vi "Pololu.Pololu Value to Deg and us Converter.vi"(7 "us to Units Mult":dbl=4.0, 9 "Pololu Value":u16, 11 "Range Info":T1={"Min us"=500.0, "Max us"=2500.0, "Min deg"=0.0, "Max deg"=270.0, "LStopDeg"=0.0, "UStopDeg"=270.0}) -> (1 "Pos (Deg)":dbl max=270.0, 3 "Pos (us)":dbl max=270.0)   [LabVIEW 2018]
uses:
  Pololu.Device Range Config.ctl
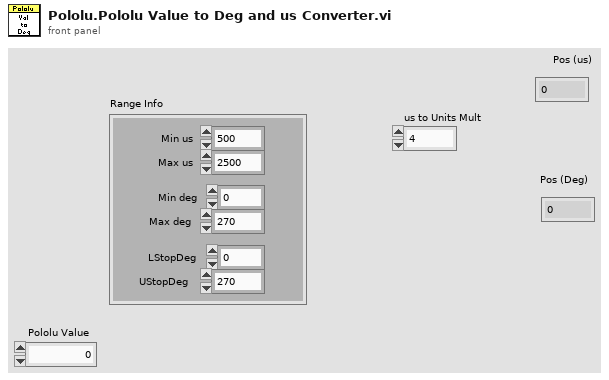
[diagram p1: front panel]
types:
  T1 = typedef "Pololu.Device Range Config.ctl" = cluster{"Min us":dbl, "Max us":dbl, "Min deg":dbl, "Max deg":dbl, "LStopDeg":dbl, "UStopDeg":dbl}
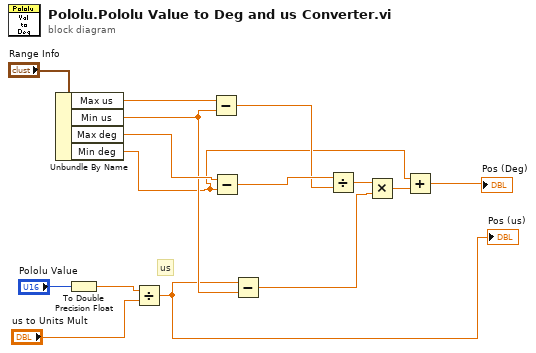
[diagram p0: block diagram]
diagram:
  # "us"
  n1 = Unbundle By Name("Range Info") -> ("Max us"=w10:dbl, "Min us"=w6:dbl, "Max deg"=w11:dbl, "Min deg"=w3:dbl)
  n2 = To Double Precision Float(number="Pololu Value") -> (double precision float=w8:dbl)
  n3 = Divide(x=w8, y="us to Units Mult") -> (x/y=w1:dbl)
  "Pos (us)" <- w1
  n4 = Subtract(x=w10, y=w6) -> (x-y=w4:dbl)
  n5 = Subtract(x=w11, y=w3) -> (x-y=w5:dbl)
  n6 = Subtract(x=w1, y=w6) -> (x-y=w14:dbl)
  n7 = Divide(x=w5, y=w4) -> (x/y=w15:dbl)
  n8 = Multiply(x=w15, y=w14) -> (x*y=w13:dbl)
  n9 = Add(x=w3, y=w13) -> (x+y=→"Pos (Deg)":dbl)
